vi "interp_prelookup.vi"(10 "x":sgl[](array[numeric]), 11 "X":sgl) -> (2 "data":T1, 3 "prelookup":cluster{"frac":dbl, "num":u8})   [LabVIEW 2014]
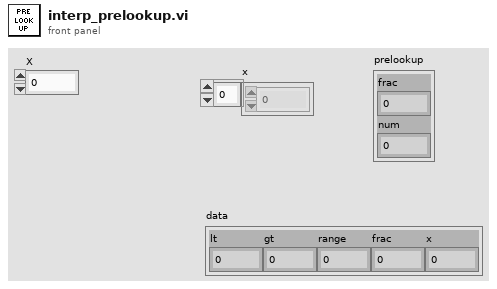
[diagram p1: front panel]
types:
  T1 = cluster{"lt":dbl, "gt":dbl, "range":dbl, "frac":dbl, "x":dbl}
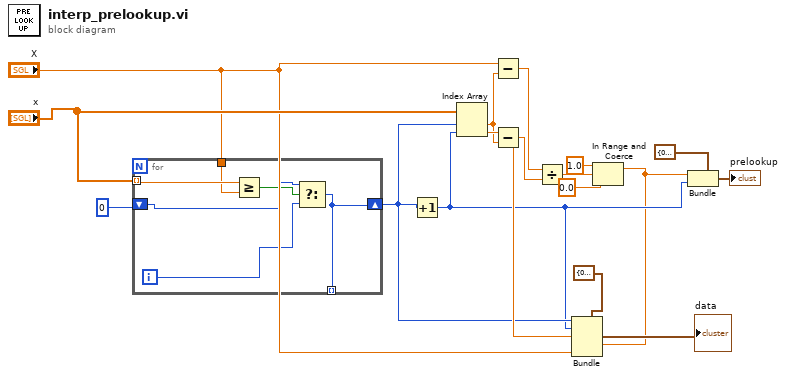
[diagram p0: block diagram]
diagram:
  n1 = for {
    tunnel: "x" -> [w23] mode=indexing
    tunnel: "X" -> [w22]
    shift-right: [w19] -> w6
    shift-left: 0 -> [w20]
    tunnel: [w19] -> _ mode=indexing
    i -> [w18]
    n2 = Greater Or Equal?(x=w23, y=w22) -> (x >= y?=w21:bool)
    n3 = Select(t=w20, s=w21, f=w18) -> (s? t:f=w19:i32)
  }
  n4 = Increment(x=w6) -> (x+1=w5:i32)
  n5 = Index Array(array="x", index #1=w6, index #2=w5) -> (element #1=w16:sgl, element #2=w17:sgl)
  n6 = Subtract(x="X", y=w16) -> (x-y=w15:sgl)
  n7 = Subtract(x=w17, y=w16) -> (x-y=w10:sgl)
  n8 = Divide(x=w15, y=w10) -> (x/y=w4:sgl)
  n9 = In Range and Coerce(upper limit=1.0, x=w4, lower limit=0.0) -> (coerced(x)=w3:dbl)  [unwired: 1 out]
  n10 = Bundle(cluster=T1 {"lt"=0.0, "gt"=0.0, "range"=0.0, "frac"=0.0, "x"=0.0} ("data"), "lt"=w6, "gt"=w5, "range"=w10, "frac"=w3, "x"="X") -> (→"data":T1)
  n11 = Bundle(cluster=cluster{"frac":dbl, "num":u8} {"frac"=0.0, "num"=0} ("prelookup"), "frac"=w3, "num"=w5) -> (→"prelookup":cluster{"frac":dbl, "num":u8})
